vi "notif_write.vi"(8 "error in (no error)":errorcluster, 11 "notification":bool) -> (0 "error out":errorcluster)   [LabVIEW 2020]
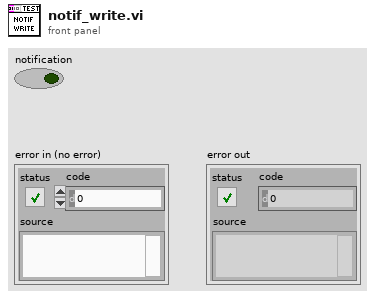
[diagram p1: front panel]
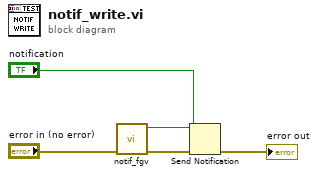
[diagram p0: block diagram]
diagram:
  n1 = call "notif_fgv.vi"("error in (no error)"="error in (no error)") -> ("error out"=w4:errorcluster, "notifier out"=w2:refnum<notifier>)  [unwired: 9 in]
  n2 = Send Notification(notification="notification", notifier=w2, error in (no error)=w4) -> (error out=→"error out":errorcluster)  [unwired: 1 out]
